vi "Exec Query.vi"(6 "scripts":string, 8 "error in":errorcluster, 11 "orm in":refnum<class "LV-ORM.lvclass">) -> (0 "error out":errorcluster, 3 "orm out":refnum<class "LV-ORM.lvclass">)   [LabVIEW 2018, in "LV-ORM.lvclass"]
uses:
  LV-ORM.lvclass
  LV-ORM.lvclass/LV-ORM.ctl
  <vilib>/addons/database/Connection.llb/Conn Execute.vi
  <vilib>/addons/database/Recordset.llb/Rec Destroy - Connection.vi
  <vilib>/addons/database/NI_Database_API.lvlib
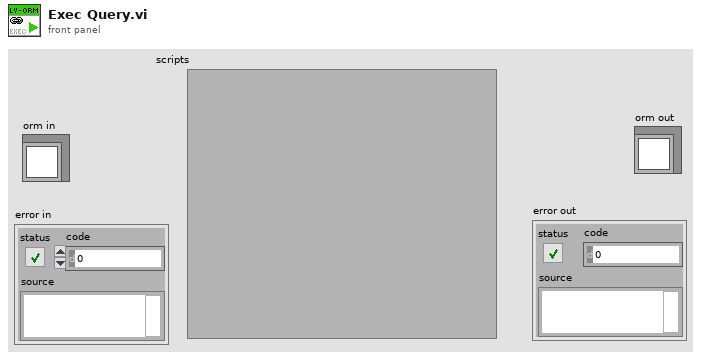
[diagram p1: front panel]
types:
  T1 = typedef "NI_Database_API.lvlib/Conn ObjectReference.ctl" = refnum<k1>
  T2 = typedef "NI_Database_API.lvlib/Rec ObjectReference.ctl" = refnum<k1>
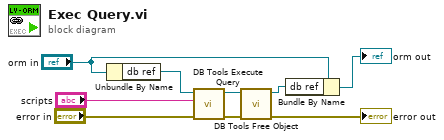
[diagram p0: block diagram]
diagram:
  n1 = Unbundle By Name("orm in") -> ("db ref"=w4:T1)
  n2 = call-poly <vilib>:"DB Tools Execute Query.vi"("error in (no error)"="error in", "SQL query"="scripts", "connection reference"=w4) -> ("error out"=w5:errorcluster, "recordset reference"=w6:T2)  [unwired: 5 in]
  n3 = call-poly <vilib>:"DB Tools Free Object.vi"("error in (no error)"=w5, "recordset reference"=w6) -> ("error out"=→"error out":errorcluster, "connection reference"=w3:T1)  [unwired: 8 in]
  n4 = Bundle By Name(cluster="orm in", "db ref"=w3) -> (→"orm out":refnum<class "LV-ORM.lvclass">)
